vi "Stop Logging.vi"(8 "error in":errorcluster, 10 "gameStatus":T1 {"gameState" items=["Start", "Pause", "Stop", "Close"]}, 11 "module reference in":T2) -> (0 "error out":errorcluster, 3 "module reference out":T2)   [LabVIEW 2017, in "WinHost.lvlib"]
uses:
  WinHost.lvlib
  Private TypeDefs/Module Reference.ctl
  Global TypeDefs/Registered Modules.ctl
  Private TypeDefs/Module Queues.ctl
  Private TypeDefs/Message Queue Element.ctl
  Public TypeDefs/Messages.ctl
  Private TypeDefs/STM Queue Element.ctl
  Private TypeDefs/Module Notifiers.ctl
  Private TypeDefs/Dummy Notifier.ctl
  Game/Libraries/TypeDefs/ClientStatusData.ctl
  Game/Libraries/GameComms.lvlib
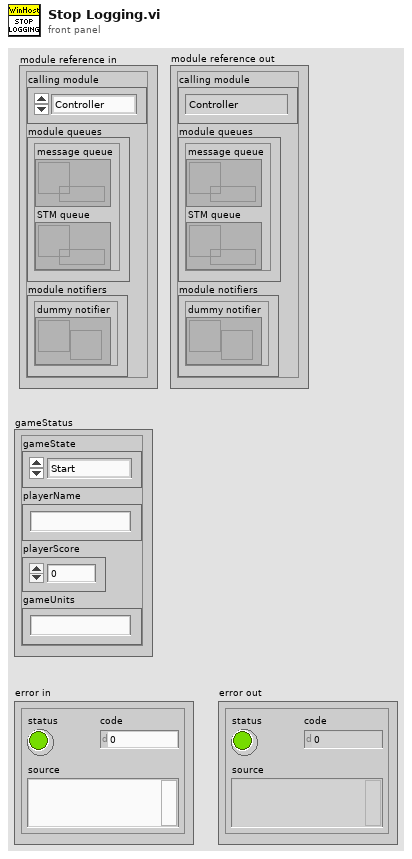
[diagram p1: front panel]
types:
  T1 = typedef "Game.lvlib/GameComms.lvlib/ClientStatusData.ctl" = cluster{"gameState":u16, "playerName":string, "playerScore":dbl, "gameUnits":string}
  T2 = typedef "WinHost.lvlib/Module Reference.ctl" = cluster{"calling module":T3, "module queues":T4, "module notifiers":T5}
  T3 = typedef "Registered Modules.ctl" = enum16{"Controller", "DAQ", "Error Handler", "Game", "myPAM", "WinHost", "Logger"}
  T4 = typedef "WinHost.lvlib/Module Queues.ctl" = cluster{"message queue":refnum<queue>, "STM queue":refnum<queue>}
  T5 = typedef "WinHost.lvlib/Module Notifiers.ctl" = cluster{"dummy notifier":refnum<notifier>}
  T6 = typedef "WinHost.lvlib/STM Queue Element.ctl" = cluster{"name":string, "data":string, "stop":bool}
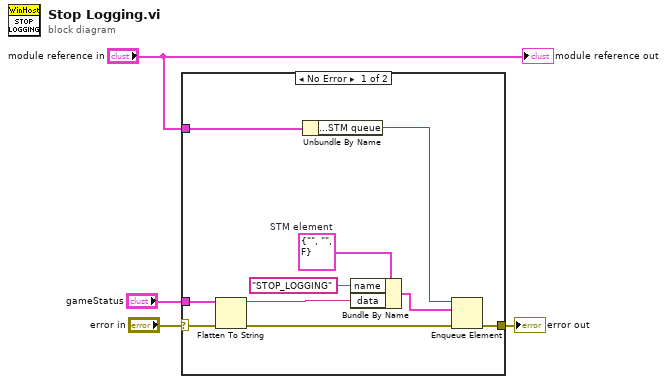
[diagram p0: block diagram]
diagram:
  n1 = case shown="No Error" "error in" {
    selector: "error in" -> [w8 w15]
    tunnel: [w13 w15] -> w4
    tunnel: "module reference in" -> [w14 _]
    tunnel: "gameStatus" -> [w6 _]
    frame No Error {
      w11 = T6 {"name"="", "data"="", "stop"=FALSE}  # STM element
      n2 = Flatten To String(anything=w6, error in (no error)=w8) -> (data string=w5:string, error out=w7:errorcluster)  [unwired: 2 in, 1 out]
      n3 = Unbundle By Name(w14) -> ("module queues.STM queue"=w12:refnum<queue>)
      n4 = Bundle By Name(cluster=w11, "name"="STOP_LOGGING", "data"=w5) -> (w10:T6)
      n5 = Enqueue Element(queue=w12, element=w10, error in (no error)=w7) -> (error out=w13:errorcluster)  [unwired: 1 in, 2 out]
    }
    frame Error {
    }
  }
  "error out" <- w4
  "module reference out" <- "module reference in"
